vi "getResponse.vi"(8 "error in (no error)":errorcluster, 9 "Function":u8, 10 "Address":u8, 11 "Mockbus in":refnum<class "Mockbus.lvclass">) -> (0 "error out":errorcluster, 2 "Frame":T1 {"Data" format="%02x"}, 3 "Mockbus out":refnum<class "Mockbus.lvclass">)   [LabVIEW 2015, in "Mockbus.lvclass"]
uses:
  Mockbus.lvclass
  Typedefs/Frame.ctl
  Mockbus.lvclass/Mockbus.ctl
  Utilities/FrameBuilder/FrameBuilder.lvclass
  Typedefs/RTTypeDefs.lvlib
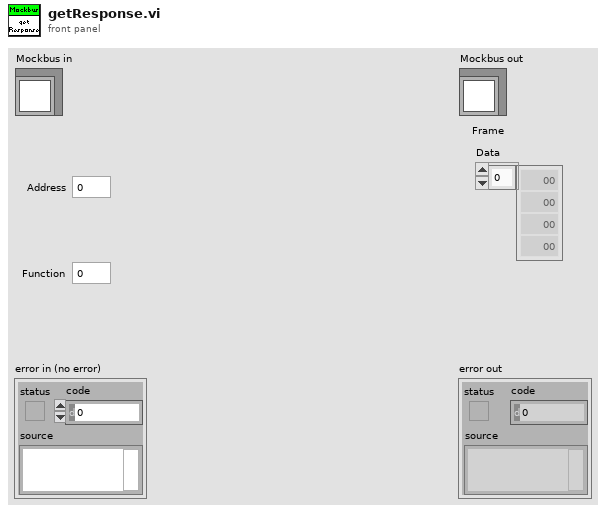
[diagram p1: front panel]
types:
  T1 = typedef "RTTypeDefs.lvlib/Frame.ctl" = cluster{"Data":u8[]}
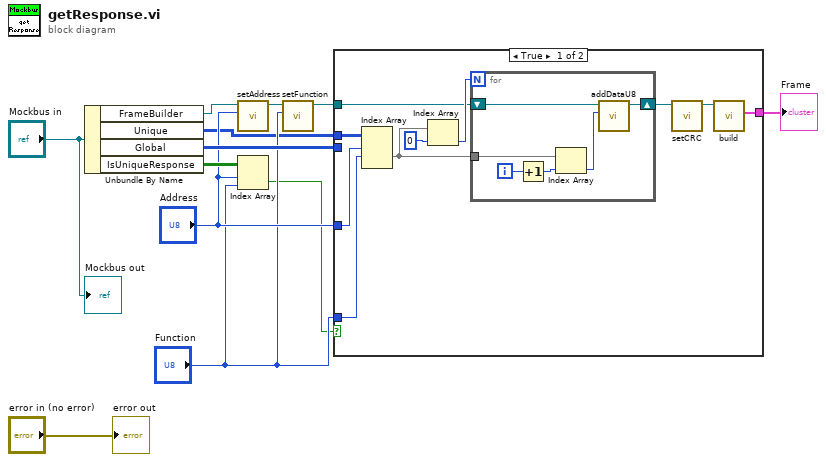
[diagram p0: block diagram]
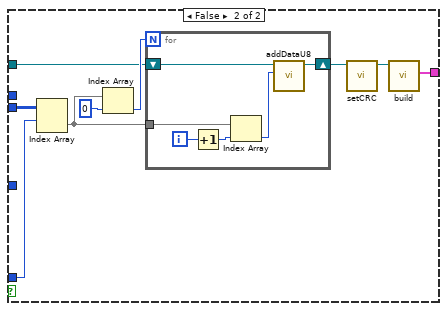
[diagram p2: hidden frame]
diagram:
  n1 = Unbundle By Name("Mockbus in") -> ("FrameBuilder"=w1:refnum<class "FrameBuilder.lvclass">, "Unique"=w5:u8[][][], "Global"=w12:u8[][], "IsUniqueResponse"=w9:bool[][])
  n2 = call "setAddress.vi"("Address"="Address", "FrameBuilder in"=w1) -> ("FrameBuilder out"=w4:refnum<class "FrameBuilder.lvclass">)  [unwired: 8 in, 1 out]
  n3 = Index Array(array=w9, index (row)="Address", index (col)="Function") -> (element=w6:bool)
  n4 = call "setFunction.vi"("Function"="Function", "FrameBuilder in"=w4) -> ("FrameBuilder out"=w3:refnum<class "FrameBuilder.lvclass">)  [unwired: 8 in, 1 out]
  n5 = case shown="True" w6 {
    tunnel: w12 -> [_ w37]
    tunnel: "Function" -> [w21 w33]
    tunnel: w5 -> [w22 _]
    tunnel: "Address" -> [w17 _]
    tunnel: w3 -> [w16 w32]
    tunnel: [w13 w29] -> w2
    frame True {
      n6 = Index Array(array=w22, index (dim 0)=w17, index (dim 1)=w21) -> (element=w18:u8[])  [unwired: 1 in]
      n7 = Index Array(array=w18, index=0) -> (element=w19:u8)
      n8 = for {
        N: w19 -> [_]
        tunnel: w18 -> [w28]
        shift-right: [w23] -> w15
        shift-left: w16 -> [w24]
        i -> [w27]
        n9 = Increment(x=w27) -> (x+1=w26:i32)
        n10 = Index Array(array=w28, index=w26) -> (element=w25:u8)
        n11 = call "addDataU8.vi"("Data"=w25, "FrameBuilder in"=w24) -> ("FrameBuilder out"=w23:refnum<class "FrameBuilder.lvclass">)  [unwired: 8 in, 1 out]
      }
      n12 = call "setCRC.vi"("FrameBuilder in"=w15) -> ("FrameBuilder out"=w14:refnum<class "FrameBuilder.lvclass">)  [unwired: 9 in, 1 out]
      n13 = call "build.vi"("FrameBuilder in"=w14) -> ("Frame"=w13:T1)  [unwired: 8 in, 2 out]
    }
    frame False {
      n14 = Index Array(array=w37, index (row)=w33) -> (element=w34:u8[])  [unwired: 1 in]
      n15 = Index Array(array=w34, index=0) -> (element=w35:u8)
      n16 = for {
        N: w35 -> [_]
        tunnel: w34 -> [w41]
        shift-right: [w38] -> w31
        shift-left: w32 -> [w39]
        i -> [w43]
        n17 = Increment(x=w43) -> (x+1=w42:i32)
        n18 = Index Array(array=w41, index=w42) -> (element=w40:u8)
        n19 = call "addDataU8.vi"("Data"=w40, "FrameBuilder in"=w39) -> ("FrameBuilder out"=w38:refnum<class "FrameBuilder.lvclass">)  [unwired: 8 in, 1 out]
      }
      n20 = call "setCRC.vi"("FrameBuilder in"=w31) -> ("FrameBuilder out"=w30:refnum<class "FrameBuilder.lvclass">)  [unwired: 9 in, 1 out]
      n21 = call "build.vi"("FrameBuilder in"=w30) -> ("Frame"=w29:T1)  [unwired: 8 in, 2 out]
    }
  }
  "Frame" <- w2
  "error out" <- "error in (no error)"
  "Mockbus out" <- "Mockbus in"
